vi "FYP_VI_MIDI_DeviceConfig.vi"() -> (2 "DeviceIdOut":u32)   [LabVIEW 2013]
panel:
  in  "MIDI Device ID :":u32
  in  "stop":bool
  in  "Blank Button":bool
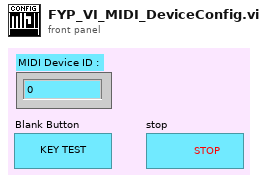
[diagram p1: front panel]
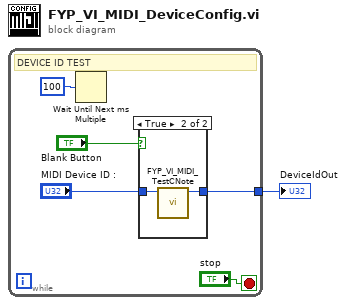
[diagram p0: block diagram]
diagram:
  n1 = while {
    tunnel: [w3] -> w1
    stop <- "stop" stop-if-true
    # "DEVICE ID TEST"
    n2 = Wait Until Next ms Multiple(millisecond multiple=u32 100) -> ()  [unwired: 1 out]
    n3 = case shown="True" "Blank Button" {
      tunnel: "MIDI Device ID :" -> [w7 w9]
      tunnel: [w7 w8] -> w3
      frame False {
      }
      frame True {
        n4 = call "FYP_VI_MIDI_TestCNote.vi"("deviceID"=w9) -> ("DeviceIdOut"=w8:u32)  [unwired: 6 in]
      }
    }
  }
  "DeviceIdOut" <- w1
